vi "RegisterMap_TrimReg.vi"(11 "Register RegMap Data IN":string[](array[string])) -> (3 "Register RegMap Data OUT":string[](array[string]))   [LabVIEW 2010]
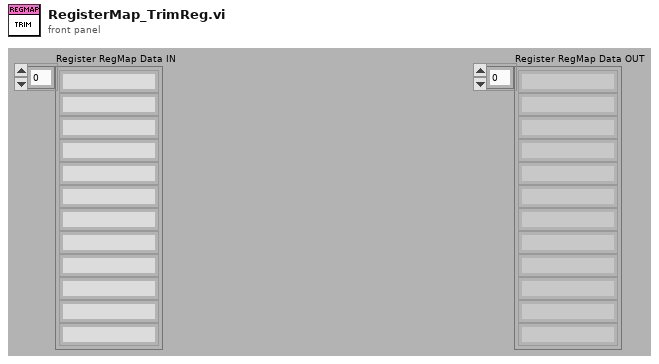
[diagram p1: front panel]
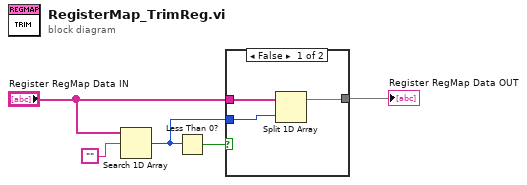
[diagram p0: block diagram]
diagram:
  n1 = Search 1D Array(1D array="Register RegMap Data IN", element="") -> (index of element=w2:i32)  [unwired: 1 out]
  n2 = Less Than 0?(x=w2) -> (x < 0?=w5:bool)
  n3 = case shown="False" w5 {
    tunnel: [w6 w9] -> w3
    tunnel: "Register RegMap Data IN" -> [w8 w9]
    tunnel: w2 -> [w7 _]
    frame False {
      n4 = Split 1D Array(array=w8, index=w7) -> (first subarray=w6:string[])  [unwired: 1 out]
    }
    frame True {
    }
  }
  "Register RegMap Data OUT" <- w3
